vi "Get Records.vi"(8 "error in (no error)":errorcluster, 10 "Records":T1 {"Step Duration" format="%#_5f"}, 11 "Car Wash Controller Actor in":refnum<class "Car Wash Controller Actor.lvclass">) -> (0 "error out":errorcluster, 3 "Car Wash Controller Actor out":refnum<class "Car Wash Controller Actor.lvclass">)   [LabVIEW 2019, in "Car Wash Controller Actor.lvlib" / "Car Wash Controller Actor.lvclass"]
uses:
  Car Wash Controller Actor.lvclass
  Configuration Database Actor/Configuration Database Actor/Records.ctl
  Car Wash Controller Actor.lvclass/Car Wash Controller Actor.ctl
  Simulated Wash Display Console Actor/Simulated Wash Display Console Actor Messages/Update Time Remaining Msg/Update Time Remaining Msg.lvclass/Update Time Remaining Msg.ctl
  <vilib>/ActorFramework/Message Enqueuer/Message Enqueuer.lvclass/Message Enqueuer.ctl
  <vilib>/ActorFramework/Message Enqueuer/Enqueue.vi
  Simulated Wash Display Console Actor/Simulated Wash Display Console Actor Messages/Update Time Remaining Msg/Update Time Remaining Msg.lvclass
  C:/Program Files (x86)/National Instruments/LabVIEW 2019/vi.lib/ActorFramework/Message/Message.lvclass
  <vilib>/ActorFramework/Message Priority Queue/Priority Enqueue.vi
  Configuration Database Actor/Configuration Database Actor/Sim Configuration Database Actor.lvclass
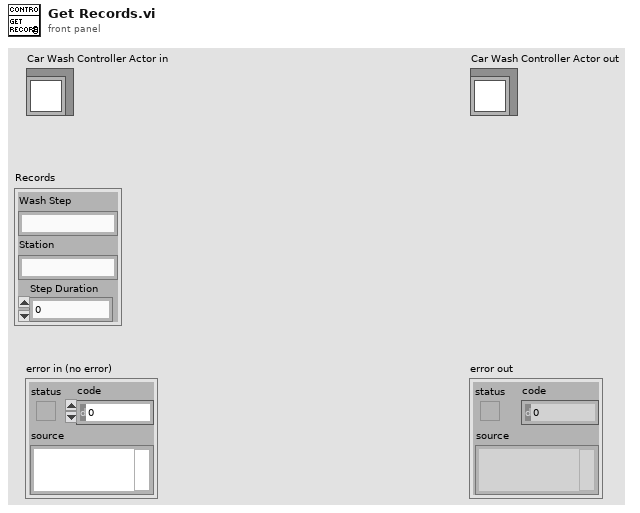
[diagram p1: front panel]
types:
  T1 = typedef "Sim Configuration Database Actor.lvlib/Sim Configuration Database Actor.lvclass/Records.ctl" = cluster{"Wash Step":string, "Station":string, "Step Duration":u32}
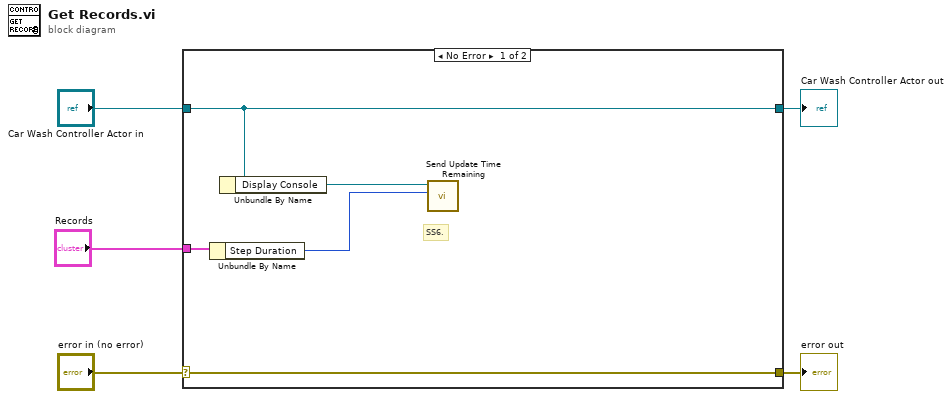
[diagram p0: block diagram]
diagram:
  n1 = case shown="No Error" "error in (no error)" {
    selector: "error in (no error)" -> [w10 w12]
    tunnel: [w10 w12] -> w4
    tunnel: [w8 w11] -> w2
    tunnel: "Car Wash Controller Actor in" -> [w8 w11]
    tunnel: "Records" -> [w9 _]
    frame No Error {
      # "SS6."
      n2 = Unbundle By Name(w9) -> ("Step Duration"=w6:u32)
      n3 = Unbundle By Name(w8) -> ("Display Console"=w7:refnum<class "Message Enqueuer.lvclass">)
      n4 = call "Send Update Time Remaining.vi"("Timing"=w6, "Message Enqueuer"=w7) -> ()  [unwired: 8 in, 2 out]
    }
    frame Error {
    }
  }
  "error out" <- w4
  "Car Wash Controller Actor out" <- w2
